vi "Copy Template Library.vi"(0 "configuration":T1, 11 "error in":errorcluster) -> (15 "error out":errorcluster)   [LabVIEW 2021, in "InstrumentStudio Plug-In Editor.lvlib"]
uses:
  InstrumentStudio Plug-In Editor.lvlib
  Data Holder.ctl
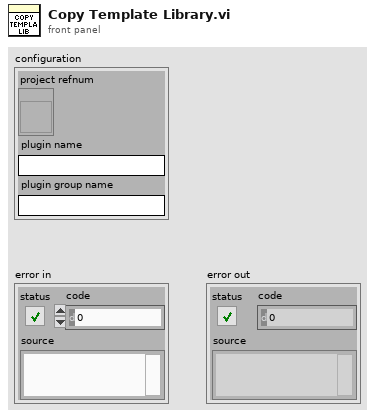
[diagram p1: front panel]
types:
  T1 = typedef "InstrumentStudio Plug-In Editor.lvlib/Data Holder.ctl" = cluster{"project refnum":refnum<vi>, "plugin name":string, "plugin group name":string}
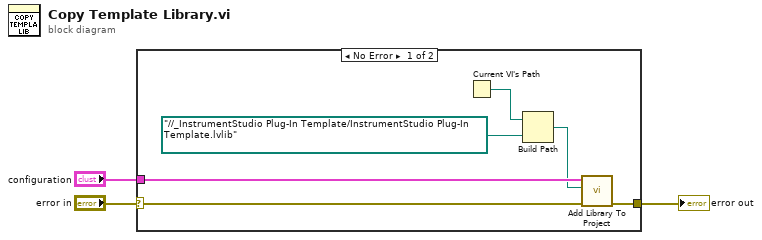
[diagram p0: block diagram]
diagram:
  n1 = case shown="No Error" "error in" {
    selector: "error in" -> [w8 w10]
    tunnel: [w9 w10] -> w1
    tunnel: "configuration" -> [w5 _]
    frame No Error {
      n2 = Current VI's Path() -> (path=w6:path)
      n3 = Build Path(base path=w6, name or relative path=path "../../_InstrumentStudio Plug-In Template/InstrumentStudio Plug-In Template.lvlib") -> (appended path=w4:path)
      n4 = call "Add Library To Project.vi"("error in"=w8, "library path"=w4, "configuration"=w5) -> ("error out"=w9:errorcluster)  [unwired: 8 in]
    }
    frame Error {
    }
  }
  "error out" <- w1
